vi "init.vi"(0 "Constant Analog Output Voltage Test in":refnum<class "Modulated Analog Output Voltage Test.lvclass">, 1 "Test Values":T1 {"Stop Value" format="%.6f"; "Start Value" format="%.6f"}, 2 "ConvertStrategy":refnum<class "IConverterStrategy.lvclass">, 3 "Tolerance":dbl format="%.3f", 4 "Samples To Average":i32, 5 "error in (no error)":errorcluster, 6 "DAQ Channel":refnum<k21>, 7 "ConfigureILCStrategy":refnum<class "IConfigureILCStrategy.lvclass">, 8 "Test Scenario":T2, 9 "ILC":refnum<class "ILC.lvclass">, 10 "Signal Name":string, 11 "Log":refnum<class "ITestLog.lvclass">, 13 "Delay Between Test Steps":u16) -> (14 "Constant Analog Output Voltage Test  out":refnum<class "Modulated Analog Output Voltage Test.lvclass">, 19 "error out":errorcluster)   [LabVIEW 2015, in "Modulated Analog Output Voltage Test.lvclass"]
uses:
  Modulated Analog Output Voltage Test.lvclass
  Model/TestLog/ITestLog/ITestLog.lvclass
  Typedefs/TestScenarioTypes.ctl
  Model/ConfigureILCStrategy/IConfigureILCStrategy/IConfigureILCStrategy.lvclass
  <userlib>/Common/ILC/ILC/ILC.lvclass
  Typedefs/Test Values.ctl
  Model/ConverterStrategy/IConverterStrategy/IConverterStrategy.lvclass
  Modulated Analog Output Voltage Test.lvclass/Modulated Analog Output Voltage Test.ctl
  Typedefs/ILCBTTypedefs.lvlib
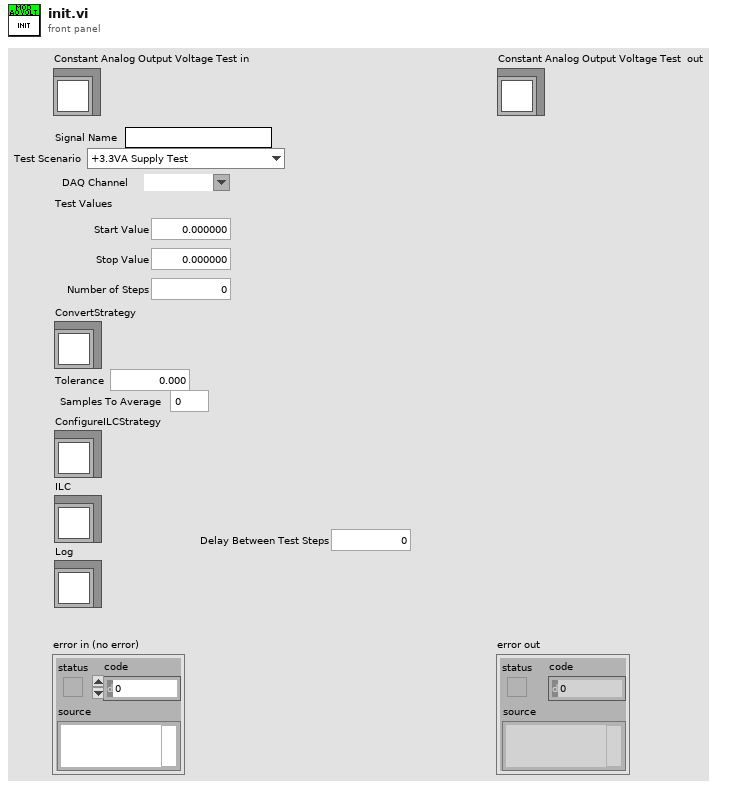
[diagram p1: front panel]
types:
  T1 = typedef "ILCBTTypedefs.lvlib/Test Values.ctl" = cluster{"Start Value":dbl, "Stop Value":dbl, "Number of Steps":u16}
  T2 = typedef "ILCBTTypedefs.lvlib/TestScenarioTypes.ctl" = enum16{"+3.3VA Supply Test", "+3.3VD Supply Test", "+5VA Supply Test", "+5VD Supply Test", "Unique ID Test", "TEDS Status Test", "LIMSW1_TTL Low Test", "LIMSW1_TTL High Test", "LIMSW2_TTL Low Test", "LIMSW2_TTL High Test", "Tachometer Low Test", "Tachometer High Test", "SSR_TTL Low Test", "SSR_TTL High Test", "SM_GPI Low Test", "SM_GPI High Test", "CW Motion Without Limit Test", "CW Motion With Limit Test", "CW Motion With Both Limits Test", "CW Motion on CCW Limit Test", "CCW Motion Without Limit Test", "CCW Motion With Limit Test", "CCW Motion With Both Limits Test", "CCW Motion on CW Limit Test", "RS232-TXD Low Test", "RS232-TXD High Test", "RS232-RTS Low Test", "RS232-RTS High Test", "RS232-RXD Low Test", "RS232-RXD High Test", "RS232-CTS Low Test", "RS232-CTS High Test", "Out_SS Low Test", "Out_SS High Test", "Out_SDI Low Test", "Out_SDI High Test", "Out_SCLK Low Test", "Out_SCLK High Test", "Reset Low Test", "Reset High Test", "1 Channel ADC Test", "3 Channel ADC Test", "5 Channel ADC Test", "Vref Test", "ROT Test", "DAC1 Test", "DAC2 Test", "DAC3 Test", "DAC4 Test", "BIAS Test", "EXC1 Test", "EXC2 Test", "EXC3 Test", "EXC4 Test"}
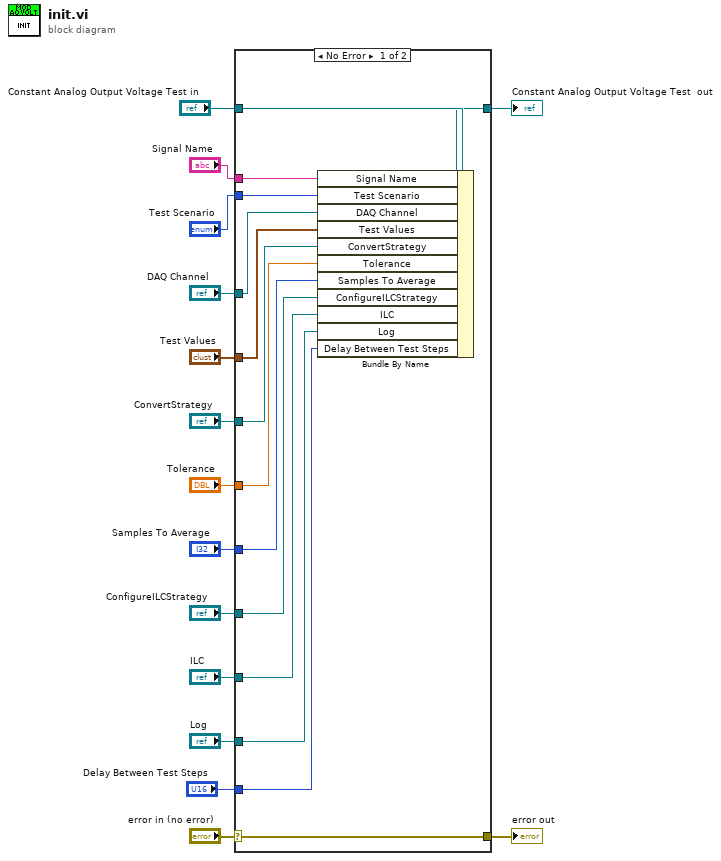
[diagram p0: block diagram]
diagram:
  n1 = case shown="No Error" "error in (no error)" {
    selector: "error in (no error)" -> [w29 w31]
    tunnel: [w29 w31] -> w14
    tunnel: [w27 w30] -> w12
    tunnel: "Constant Analog Output Voltage Test in" -> [w28 w30]
    tunnel: "Signal Name" -> [w26 _]
    tunnel: "Test Scenario" -> [w25 _]
    tunnel: "DAQ Channel" -> [w24 _]
    tunnel: "Test Values" -> [w23 _]
    tunnel: "ConvertStrategy" -> [w22 _]
    tunnel: "Tolerance" -> [w21 _]
    tunnel: "Samples To Average" -> [w20 _]
    tunnel: "ConfigureILCStrategy" -> [w19 _]
    tunnel: "ILC" -> [w18 _]
    tunnel: "Log" -> [w17 _]
    tunnel: "Delay Between Test Steps" -> [w16 _]
    frame No Error {
      n2 = Bundle By Name(cluster=w28, "Signal Name"=w26, "Test Scenario"=w25, "DAQ Channel"=w24, "Test Values"=w23, "ConvertStrategy"=w22, "Tolerance"=w21, "Samples To Average"=w20, "ConfigureILCStrategy"=w19, "ILC"=w18, "Log"=w17, "Delay Between Test Steps"=w16) -> (w27:refnum<class "Modulated Analog Output Voltage Test.lvclass">)
    }
    frame Error {
    }
  }
  "error out" <- w14
  "Constant Analog Output Voltage Test  out" <- w12
